vi "Point Cloud Analyze Test.vi"() -> ()   [LabVIEW 2018]
uses:
  Controls/cls_Point_Cloud_Data.ctl
  Controls/cls_Point_Cloud_Packet_Header.ctl
  Controls/cls_Point_Cloud_Ray_Header.ctl
  Controls/cls_Point_Cloud_Return_Data.ctl
  LiDAR.lvclass
panel:
  out "x+1":u64
  out "Reflectance A":dbl(graph) caption="Waveform Chart - Dark"
  out "Reflectance B":dbl(graph) caption="Waveform Chart - Dark"
  out "Range (m) Site B":dbl(graph) caption="Waveform Chart - Dark"
  out "Range (m) Site A":dbl(graph) caption="Waveform Chart - Dark"
  out "Return Description":T1(array[cluster])
  in  "LiDAR in":refnum<class "LiDAR.lvclass">
  out "Array":T2[](array[typedef]) {"Ray Header Data"."Return Data Array"."Reflectance" format="%.6f %"; "Ray Header Data"."Return Data Array"."Range" format="%.4f M"; "Ray Header Data"."Return Data Array"."Existence Probability" format="%.4f %"; "Ray Header Data"."Elevation" format="%.6f"; "Ray Header Data"."Azimuth" format="%.6f"}
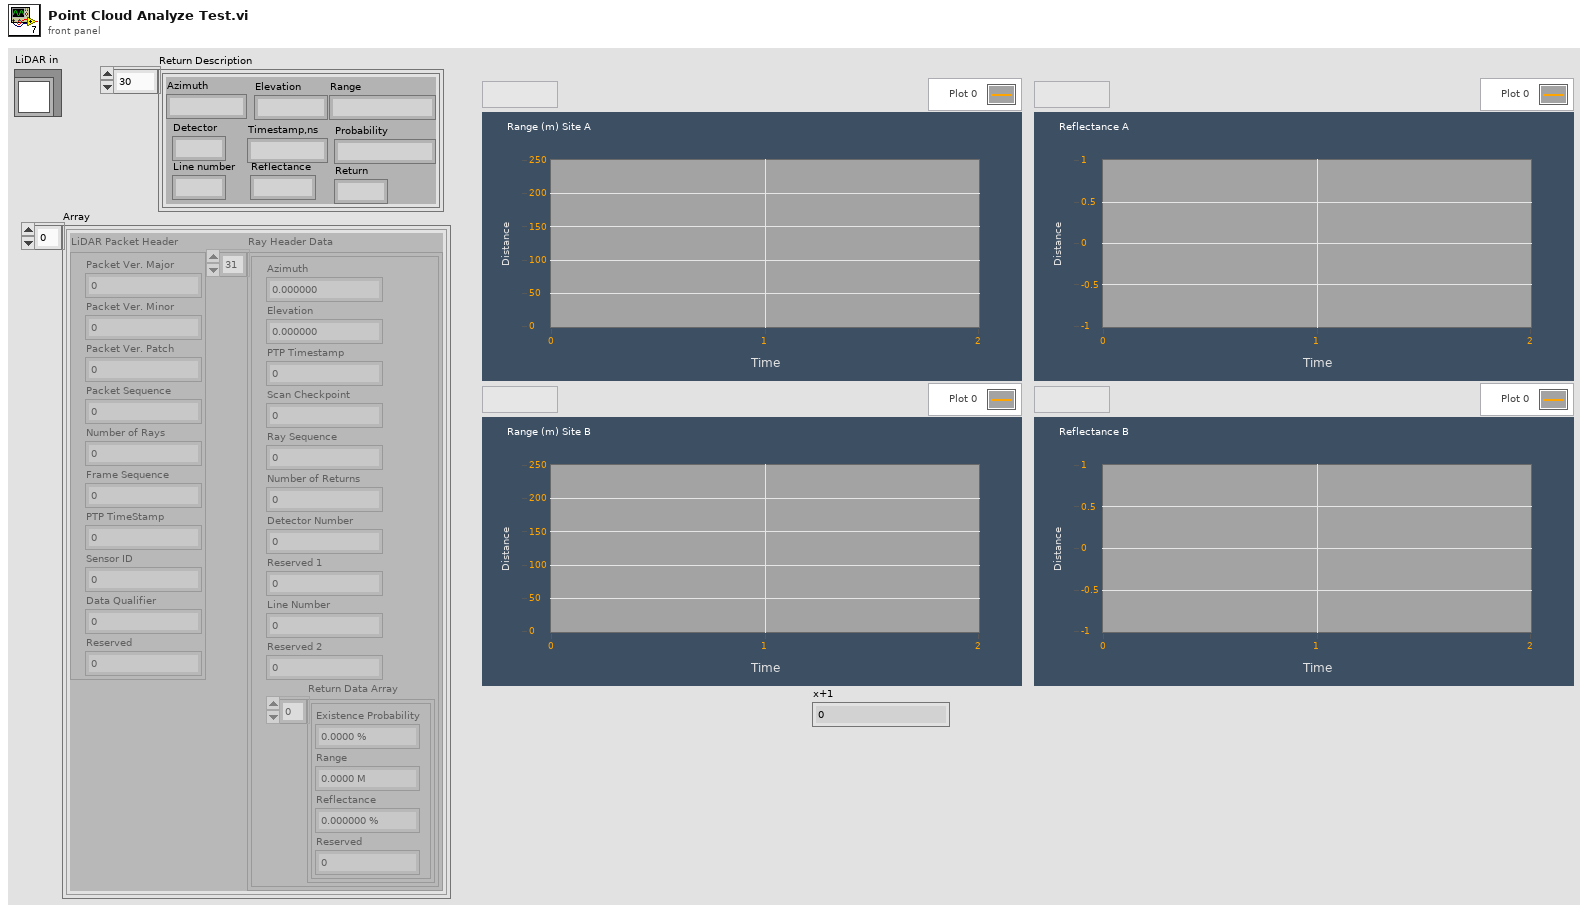
[diagram p1: front panel]
types:
  T1 = cluster{"Azimuth":dbl, "Elevation":dbl, "Timestamp,ns":u32, "Detector":i32, "Line number":u16, "Range":ext, "Probability":ext, "Reflectance":ext, "Return":ext}[]
  T2 = typedef "LiDAR.lvlib/LiDAR.lvclass/cls_Point_Cloud_Data.ctl" = cluster{"LiDAR Packet Header":T3, "Ray Header Data":T4[]}
  T3 = typedef "LiDAR.lvlib/LiDAR.lvclass/cls_Point_Cloud_Packet_Header.ctl" = cluster{"Packet Ver. Major":u8, "Packet Ver. Minor":u8, "Packet Ver. Patch":u8, "Packet Sequence":u8, "Number of Rays":u8, "Frame Sequence":u8, "PTP TimeStamp":u64, "Sensor ID":u8, "Data Qualifier":u8, "Reserved":u16}
  T4 = typedef "LiDAR.lvlib/LiDAR.lvclass/cls_Point_Cloud_Ray_Header.ctl" = cluster{"Azimuth":dbl, "Elevation":dbl, "PTP Timestamp":u32, "Scan Checkpoint":u8, "Ray Sequence":u8, "Number of Returns":u8, "Detector Number":u8, "Reserved 1":u8, "Line Number":u16, "Reserved 2":u32, "Return Data Array":T5[]}
  T5 = typedef "LiDAR.lvlib/LiDAR.lvclass/cls_Point_Cloud_Return_Data.ctl" = cluster{"Existence Probability":dbl, "Range":dbl, "Reflectance":dbl, "Reserved":u16}
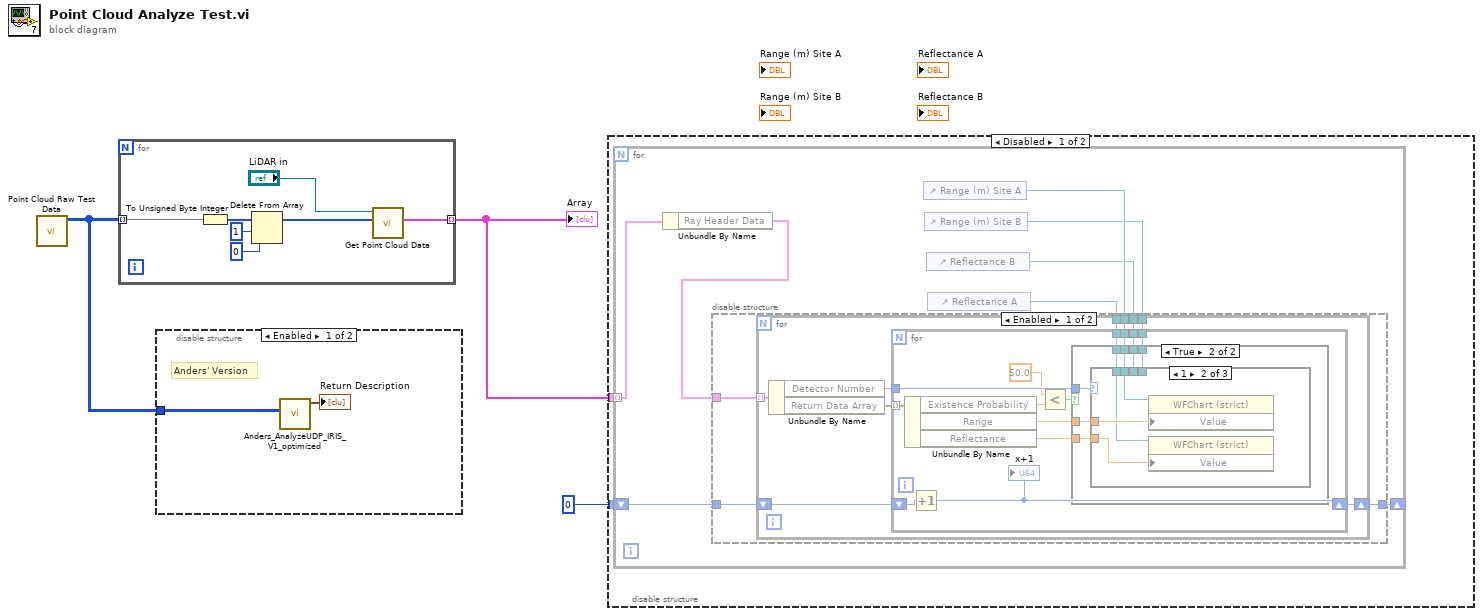
[diagram p0: block diagram]
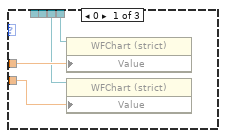
[diagram p3: hidden frame]
diagram:
  n1 = call "Point Cloud Raw Test Data.vi"() -> ("Input UDP packet array 2"=w3:i32[][])  [unwired: 11 in]
  n2 = for {
    tunnel: w3 -> [w8] mode=indexing
    tunnel: [w10] -> w2 mode=indexing
    n3 = To Unsigned Byte Integer(number=w8) -> (unsigned 8bit integer=w5:u8[])
    n4 = Delete From Array(array=w5, length=1, index=0) -> (array with subset deleted=w4:u8[])  [unwired: 1 out]
    n5 = call "Get Point Cloud Data.vi"("Test Data"=w4, "LiDAR in"="LiDAR in") -> ("Pount Cloud Data out"=w10:T2)  [unwired: 7 in, 2 out]
  }
  "Array" <- w2
  n6 = disable-structure shown="Enabled" {
    disable-tunnel: w3 -> [w12 _]
    frame Enabled {
      # "Anders' Version"
      n7 = call "Anders_AnalyzeUDP_IRIS_V1_optimized.vi"("Input UDP packet array"=w12) -> ("Return Description"=→"Return Description":T1)  [unwired: 8 in, 2 out]
    }
    frame Disabled {
    }
  }
  n8 = disable-structure shown="Disabled" {
    disable-tunnel: w2 -> [w14 _]
    disable-tunnel: u64 0 -> [w13 _]
    frame Disabled {
      n9 = for {
        tunnel: w14 -> [w18] mode=indexing
        shift-right: [w15] -> _
        shift-left: w13 -> [w16]
        n10 = Unbundle By Name(w18) -> ("Ray Header Data"=w17:T4[])
        n11 = control-ref of="Range (m) Site A"() -> (w22:refnum<vi>)
        n12 = control-ref of="Range (m) Site B"() -> (w21:refnum<vi>)
        n13 = control-ref of="Reflectance B"() -> (w20:refnum<vi>)
        n14 = control-ref of="Reflectance A"() -> (w19:refnum<vi>)
        n15 = disable-structure shown="Enabled" {
          disable-tunnel: w21 -> [w29 _]
          disable-tunnel: w20 -> [w28 _]
          disable-tunnel: w22 -> [w27 _]
          disable-tunnel: w19 -> [w26 _]
          disable-tunnel: w17 -> [w25 _]
          disable-tunnel: w16 -> [w24 _]
          disable-tunnel: [w23 _] -> w15
          frame Enabled {
            n16 = for {
              tunnel: w29 -> [w36]
              tunnel: w28 -> [w35]
              tunnel: w27 -> [w34]
              tunnel: w26 -> [w33]
              tunnel: w25 -> [w32] mode=indexing
              shift-right: [w30] -> w23
              shift-left: w24 -> [w31]
              n17 = Unbundle By Name(w32) -> ("Detector Number"=w37:u8, "Return Data Array"=w38:T5[])
              n18 = for {
                tunnel: w38 -> [w51] mode=indexing
                tunnel: w37 -> [w49]
                tunnel: w36 -> [w44]
                tunnel: w35 -> [w43]
                tunnel: w34 -> [w42]
                tunnel: w33 -> [w41]
                shift-right: [w39] -> w30
                shift-left: w31 -> [w40]
                n19 = Unbundle By Name(w51) -> ("Existence Probability"=w48:dbl, "Range"=w46:dbl, "Reflectance"=w45:dbl)
                n20 = Increment(x=w40) -> (x+1=w39:u64)
                "x+1" <- w39
                n21 = Less?(x=50.0 ("y"), y=w48) -> (x < y?=w50:bool)
                n22 = case shown="True" w50 {
                  tunnel: w49 -> [_ w58]
                  tunnel: w46 -> [_ w57]
                  tunnel: w45 -> [_ w56]
                  tunnel: w44 -> [_ w55]
                  tunnel: w43 -> [_ w54]
                  tunnel: w42 -> [_ w53]
                  tunnel: w41 -> [_ w52]
                  frame False {
                  }
                  frame True {
                    n23 = case shown="1" w58 {
                      tunnel: w57 -> [w62 w66 _]
                      tunnel: w56 -> [w61 w65 _]
                      tunnel: w55 -> [w60 _ _]
                      tunnel: w54 -> [w59 _ _]
                      tunnel: w53 -> [_ w64 _]
                      tunnel: w52 -> [_ w63 _]
                      frame 0 {
                        n24 = property class="WFChart (strict)"(reference=w60, "Value"=w62) -> ()  [unwired: 1 in, 2 out]
                        n25 = property class="WFChart (strict)"(reference=w59, "Value"=w61) -> ()  [unwired: 1 in, 2 out]
                      }
                      frame 1 {
                        n26 = property class="WFChart (strict)"(reference=w64, "Value"=w66) -> ()  [unwired: 1 in, 2 out]
                        n27 = property class="WFChart (strict)"(reference=w63, "Value"=w65) -> ()  [unwired: 1 in, 2 out]
                      }
                      frame Default {
                      }
                    }
                  }
                }
              }
            }
          }
          frame Disabled {
          }
        }
      }
    }
    frame Enabled {
    }
  }
